vi "01 LV - Offline client lifecycle.vi"() -> ()   [LabVIEW 2020]
uses:
  client/Client/Client.lvclass
panel:
  out "base url":string
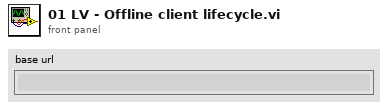
[diagram p1: front panel]
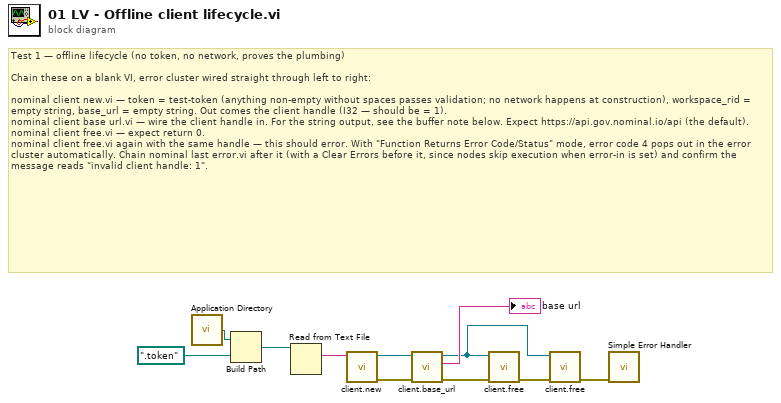
[diagram p0: block diagram]
diagram:
  # "Test 1 — offline lifecycle (no token, no network, proves the plumbing)\n\nChain these on a blank VI, error cluster wired straight through left to right:\n\nnominal client new.vi — token = test-token (anything non-empty without spaces passes validation; no network happens at construction), workspace_rid = empty string, base_url = empty string. Out comes the client handle (I32 — should be = 1).\nnominal client base url.vi — wire the client handle in. For the string output, see the buffer note below. Expect https://api.gov.nominal.io/api (the default).\nnominal client free.vi — expect return 0.\nnominal client free.vi again with the same handle — this should error. With \"Function Returns Error Code/Status\" mode, error code 4 pops out in the error cluster automatically. Chain nominal last error.vi after it (with a Clear Errors before it, since nodes skip execution when error-in is set) and confirm the message reads \"invalid client handle: 1\"."
  n1 = call <vilib>:"Application Directory.vi"() -> ("Application Directory"=w11:path)
  n2 = Build Path(base path=w11, name or relative path=path ".token") -> (appended path=w9:path)
  n3 = Read from Text File(file (use dialog)=w9) -> (text=w8:string)  [unwired: 3 in, 3 out]
  n4 = call "client.new.vi"("token"=w8) -> ("error out"=w6:errorcluster, "Client out"=w7:refnum<class "Client.lvclass">)  [unwired: 9 in]
  n5 = call "client.base_url.vi"("error in"=w6, "Client in"=w7) -> ("error out"=w5:errorcluster, "base url"=→"base url":string, "Client out"=w1:refnum<class "Client.lvclass">)  [unwired: 7 in]
  n6 = call "client.free.vi"("error in"=w5, "Client in"=w1) -> ("error out"=w3:errorcluster)  [unwired: 9 in]
  n7 = call "client.free.vi"("error in"=w3, "Client in"=w1) -> ("error out"=w2:errorcluster)  [unwired: 9 in]
  n8 = call <vilib>:"Simple Error Handler.vi"("error in (no error)"=w2) -> ()  [unwired: 4 in, 5 out]
